vi "Do Create Control.vi"(8 "error in (no error)":errorcluster, 10 "create_control Argument":T2, 11 "Data Cluster in":T1) -> (0 "error out":errorcluster, 2 "new reference":i32, 3 "Data Cluster out":T1)   [LabVIEW 2025, in "Scripting Server.lvlib"]
uses:
  Scripting Server.lvlib
  create_control Argument--cluster.ctl
  create_control (Reply Payload)--cluster.ctl
  Module Data--cluster.ctl
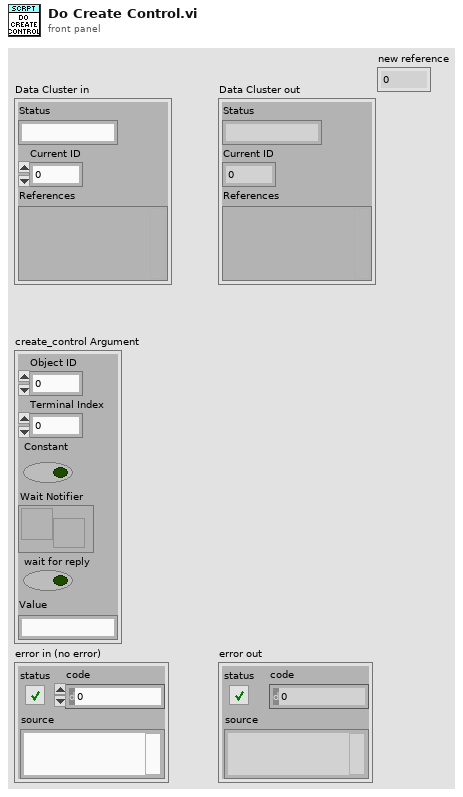
[diagram p1: front panel]
types:
  T1 = typedef "Scripting Server.lvlib/Module Data--cluster.ctl" = cluster{"Status":string, "Current ID":i32, "References":variant}
  T2 = typedef "Scripting Server.lvlib/create_control Argument--cluster.ctl" = cluster{"Object ID":i32, "Terminal Index":i32, "Constant":bool, "Wait Notifier":refnum<notifier>, "wait for reply":bool, "Value":string}
  T3 = typedef "Datatypes.ctl" = enum16{"Float", "Int", "String", "Bool", "Invalid"}
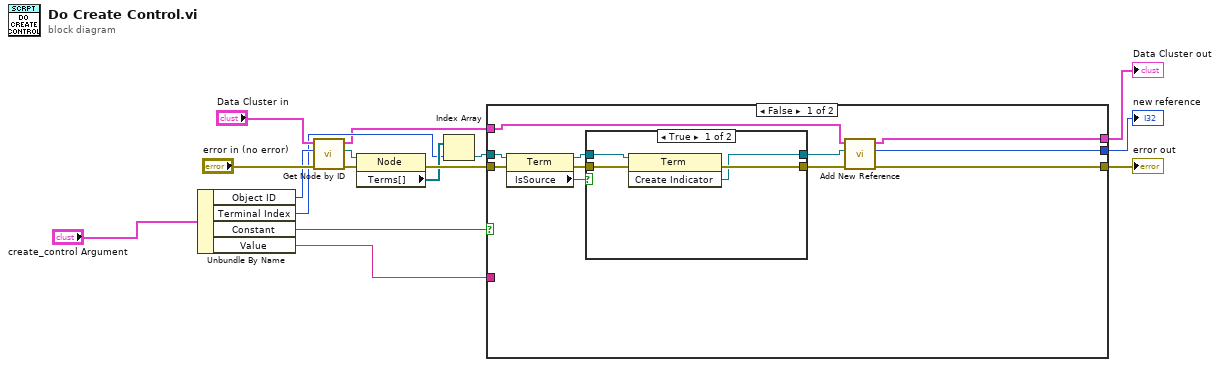
[diagram p0: block diagram]
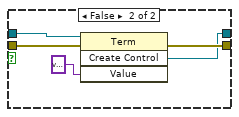
[diagram p2: hidden frame]
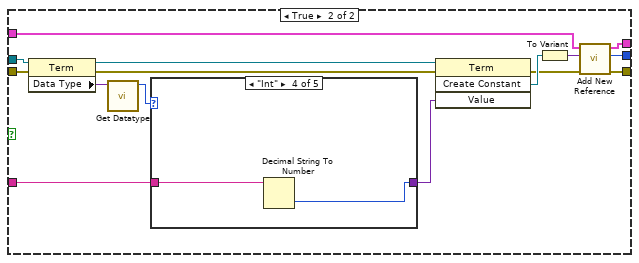
[diagram p3: hidden frame]
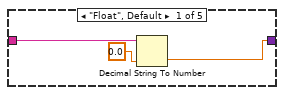
[diagram p4: hidden frame]
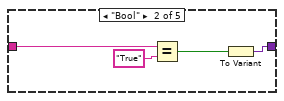
[diagram p5: hidden frame]
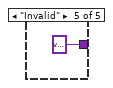
[diagram p7: hidden frame]
diagram:
  n1 = Unbundle By Name("create_control Argument") -> ("Object ID"=w12:i32, "Terminal Index"=w9:i32, "Constant"=w6:bool, "Value"=w2:string)
  n2 = call "Get Node by ID.vi"("error in (no error)"="error in (no error)", "ID"=w12, "Data Cluster in"="Data Cluster in") -> ("error out"=w13:errorcluster, "specific class reference"=w1:refnum<vi>, "Data Cluster out"=w5:T1)  [unwired: 6 in]
  n3 = property class="Node"(reference=w1, error in=w13) -> (error out=w11:errorcluster, "Terms[]"=w10:refnum<vi>[])  [unwired: 1 out]
  n4 = Index Array(array=w10, index=w9) -> (element=w7:refnum<vi>)
  n5 = case shown="False" w6 {
    tunnel: w11 -> [w27 w51]
    tunnel: [w21 w45] -> w8
    tunnel: w7 -> [w25 w42]
    tunnel: [w20 w50] -> w4
    tunnel: w5 -> [w19 w49]
    tunnel: [w17 w44] -> w3
    tunnel: w2 -> [_ w39]
    frame False {
      n6 = property class="Term"(reference=w25, error in=w27) -> (reference out=w24:refnum<vi>, error out=w26:errorcluster, "IsSource"=w23:bool)
      n7 = case shown="True" w23 {
        tunnel: [w31 w36] -> w22
        tunnel: w26 -> [w30 w35]
        tunnel: w24 -> [w29 w34]
        tunnel: [w28 w33] -> w18
        frame True {
          n8 = invoke class="Term" method="Create Indicator"(reference=w29, error in=w30) -> (error out=w31:errorcluster, "Create Indicator"=w28:refnum<vi>)  [unwired: 1 in, 1 out]
        }
        frame False {
          n9 = invoke class="Term" method="Create Control"(reference=w34, error in=w35, "Value"=variant) -> (error out=w36:errorcluster, "Create Control"=w33:refnum<vi>)  [unwired: 1 in, 2 out]
        }
      }
      n10 = call "Add New Reference.vi"("error in (no error)"=w22, "Variant"=w18, "Data Cluster in"=w19) -> ("error out"=w21:errorcluster, "new reference"=w17:i32, "Data Cluster out 2"=w20:T1)  [unwired: 6 in]
    }
    frame True {
      n11 = property class="Term"(reference=w42, error in=w51) -> (reference out=w41:refnum<vi>, error out=w43:errorcluster, "Data Type"=w40:variant)
      n12 = call "Get Datatype.vi"("Value"=w40) -> ("datatypes"=w37:T3)  [unwired: 10 in]
      n13 = case shown="\"Int\"" w37 {
        tunnel: w39 -> [w54 w57 w59 w61 _]
        tunnel: [w52 w55 w59 w60 variant ("Variant")] -> w38
        frame "Float", Default {
          n14 = Decimal String To Number(string=w54, default (0L)=0.0 ("default (0 I32)")) -> (number=w52:dbl)  [unwired: 1 in, 1 out]
        }
        frame "Bool" {
          n15 = Equal?(x=w57, y="True") -> (x = y?=w56:bool)
          n16 = To Variant(anything=w56) -> (Variant=w55:variant)
        }
        frame "String" {
        }
        frame "Int" {
          n17 = Decimal String To Number(string=w61) -> (number=w60:i32)  [unwired: 2 in, 1 out]
        }
        frame "Invalid" {
        }
      }
      n18 = invoke class="Term" method="Create Constant"(reference=w41, error in=w43, "Value"=w38) -> (error out=w46:errorcluster, "Create Constant"=w48:refnum<vi>)  [unwired: 1 in, 2 out]
      n19 = To Variant(anything=w48) -> (Variant=w47:variant)
      n20 = call "Add New Reference.vi"("error in (no error)"=w46, "Variant"=w47, "Data Cluster in"=w49) -> ("error out"=w45:errorcluster, "new reference"=w44:i32, "Data Cluster out 2"=w50:T1)  [unwired: 6 in]
    }
  }
  "Data Cluster out" <- w4
  "error out" <- w8
  "new reference" <- w3
